vi "uArm_SendGCode.vi"() -> ()   [LabVIEW 2017]
panel:
  in  "OK Button":bool
  in  "stop":bool
  in  "error in":errorcluster
  out "error out":errorcluster
  in  "VISA Refnum in":refnum<visa-resource-name>="ASRL1::INSTR"
  in  "Write Buffer":string="G91 G0 X1\n"
  out "read buffer":string
  in  "Step Size":dbl=1.0
  in  "Speed":dbl=8000.0
  in  "X":dbl
  in  "Y":dbl
  in  "Z":dbl
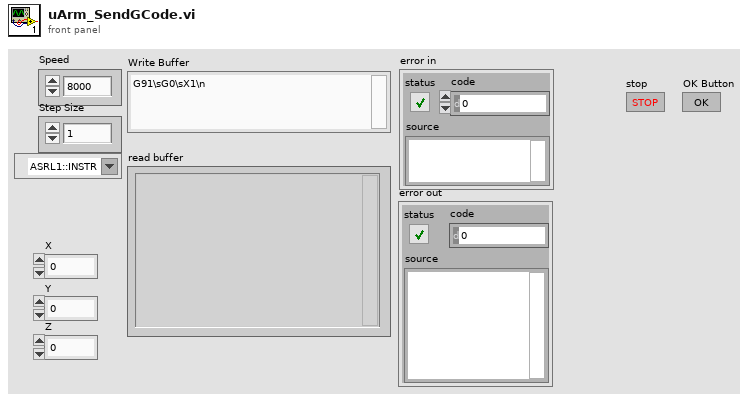
[diagram p1: front panel]
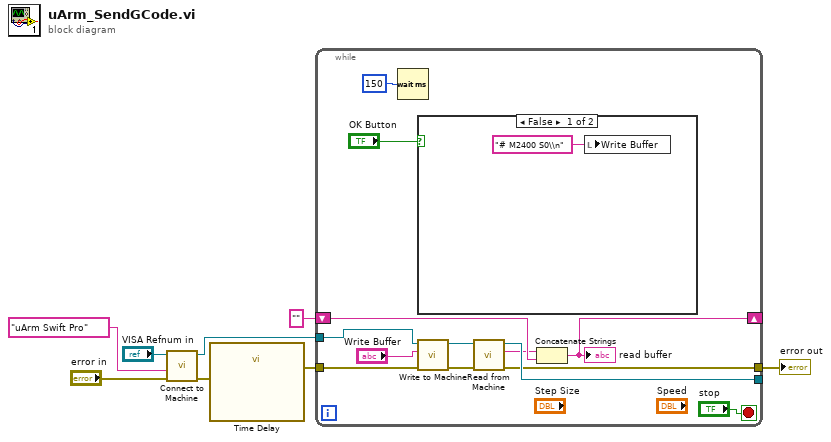
[diagram p0: block diagram]
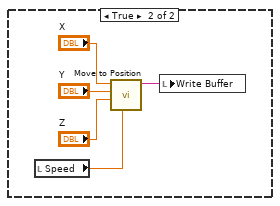
[diagram p2: hidden frame]
diagram:
  n1 = call "Connect to Machine .vi"(8:"error in", "Firmware"="uArm Swift Pro", "Machine In"="VISA Refnum in") -> ("error out"=w4:errorcluster, "Machine Out"=w7:refnum<visa-resource-name>)  [unwired: 6 in, 1 out]
  n2 = call "Time Delay"("error in (no error)"=w4) -> ("error out"=w5:errorcluster)  [unwired: 10 in]
  n3 = while {
    tunnel: w7 -> [w16]
    tunnel: w5 -> [w12]
    shift-right: [w13] -> _
    shift-left: "" -> [w15]
    tunnel: [w18] -> _
    tunnel: [w11] -> w2
    stop <- "stop" stop-if-true
    n4 = Wait (ms)(milliseconds to wait=u32 150) -> ()  [unwired: 1 out]
    n5 = case shown="False" "OK Button" {
      frame False {
        n6 = local write "Write Buffer"("# M2400 S0\\n") -> ()
      }
      frame True {
        n7 = local read "Speed"() -> (w27:dbl)
        n8 = call "Move to Position.vi"("Speed"=w27, "Z-Position"="Z", "Y-Position"="Y", "X-Position"="X") -> ("G-Code String"=w26:string)  [unwired: 7 in]
        n9 = local write "Write Buffer"(w26) -> ()
      }
    }
    n10 = call "Write to Machine .vi"("error in (no error)"=w12, "G-Code String In"="Write Buffer", "Machine In"=w16) -> ("error out"=w19:errorcluster, "Machine Out"=w20:refnum<visa-resource-name>)  [unwired: 7 in]
    n11 = call "Read from Machine.vi"("error in (no error)"=w19, "Machine In"=w20) -> ("error out"=w11:errorcluster, "read buffer"=w14:string, "Machine Out"=w18:refnum<visa-resource-name>)  [unwired: 7 in]
    n12 = Concatenate Strings(w14, w15) -> (w13:string)
    "read buffer" <- w13
  }
  "error out" <- w2
